vi "vizualization.vi"() -> ()   [LabVIEW 2020]
uses:
  globalVariables.vi
panel:
  out "Velocity of the rover's right-side wheels":dbl(graph)
  out "Scientific notation":dbl
  out "Rover wheel velocity on the right side":string
  out "Rover wheel velocity on the left side":string
  out "Scientific notation 2":dbl
  out "Velocity of the rover's left-side wheels":dbl(graph)
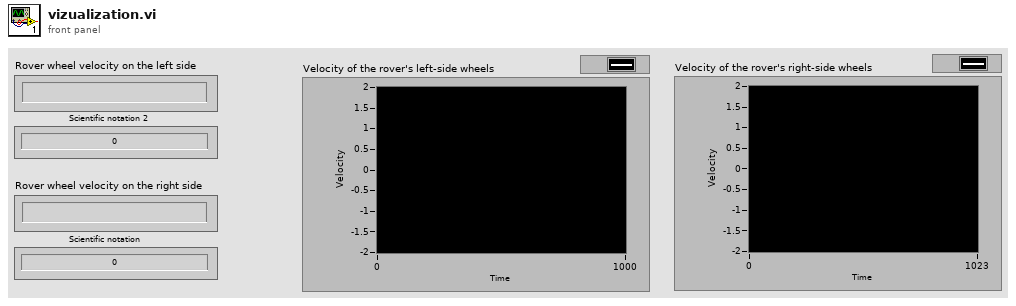
[diagram p1: front panel]
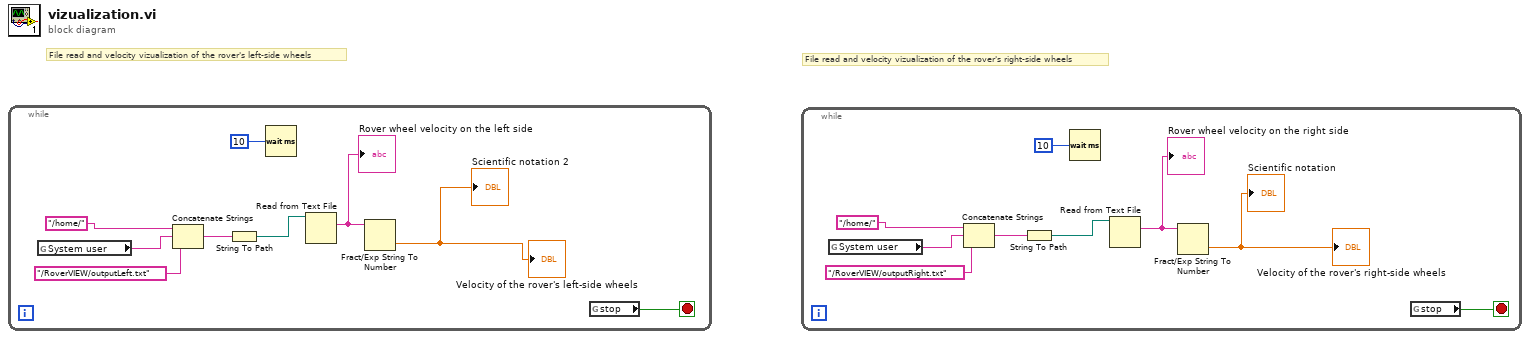
[diagram p0: block diagram]
diagram:
  # "File read and velocity vizualization of the rover's right-side wheels"
  # "File read and velocity vizualization of the rover's left-side wheels"
  n1 = while {
    stop <- w1 stop-if-true
    n2 = global read "globalVariables.vi" "System user"() -> (w6:string)
    n3 = Concatenate Strings("/home/", w6, "/RoverVIEW/outputLeft.txt") -> (w4:string)
    n4 = String To Path(string=w4) -> (path=w8:path)
    n5 = Wait (ms)(milliseconds to wait=u32 10) -> ()  [unwired: 1 out]
    n6 = Read from Text File(file (use dialog)=w8) -> (text=w3:string)  [unwired: 3 in, 3 out]
    "Rover wheel velocity on the left side" <- w3
    n7 = Fract/Exp String To Number(string=w3) -> (number=→"Scientific notation 2" →"Velocity of the rover's left-side wheels":dbl)  [unwired: 3 in, 1 out]
    n8 = global read "globalVariables.vi" "stop"() -> (w1:bool)
  }
  n9 = while {
    stop <- w10 stop-if-true
    n10 = global read "globalVariables.vi" "System user"() -> (w16:string)
    n11 = Concatenate Strings("/home/", w16, "/RoverVIEW/outputRight.txt") -> (w14:string)
    n12 = String To Path(string=w14) -> (path=w13:path)
    n13 = Wait (ms)(milliseconds to wait=u32 10) -> ()  [unwired: 1 out]
    n14 = Read from Text File(file (use dialog)=w13) -> (text=w11:string)  [unwired: 3 in, 3 out]
    "Rover wheel velocity on the right side" <- w11
    n15 = Fract/Exp String To Number(string=w11) -> (number=→"Velocity of the rover's right-side wheels" →"Scientific notation":dbl)  [unwired: 3 in, 1 out]
    n16 = global read "globalVariables.vi" "stop"() -> (w10:bool)
  }
